vi "time2mm_delta.vi"(3 "Delta time":dbl) -> (0 "Delta position (mm)":dbl)   [LabVIEW 2020]
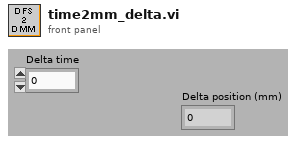
[diagram p1: front panel]
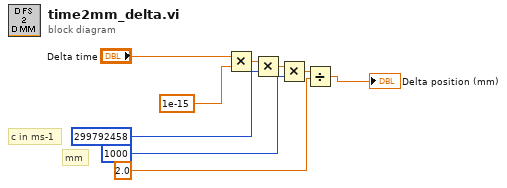
[diagram p0: block diagram]
diagram:
  # "mm"
  # "c in ms-1"
  n1 = Multiply(x="Delta time", y=1e-15) -> (x*y=w2:dbl)
  n2 = Multiply(x=w2, y=299792458) -> (x*y=w4:dbl)
  n3 = Multiply(x=w4, y=1000) -> (x*y=w6:dbl)
  n4 = Divide(x=w6, y=2.0) -> (x/y=→"Delta position (mm)":dbl)
